vi "ReadAsyncErrorHandling.vi"(8 "ErrorIn":errorcluster, 11 "YActorIn":refnum<class "YActor.lvclass">) -> (0 "ErrorOut":errorcluster, 2 "AsyncErrorHandling":T1, 3 "YActorOut":refnum<class "YActor.lvclass">)   [LabVIEW 2021, in "YActor.lvclass"]
uses:
  YActor.lvclass
  AsyncErrorHandling.ctl
  YActor.lvclass/YActor.ctl
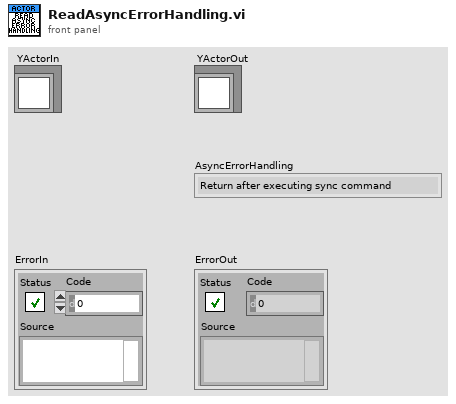
[diagram p1: front panel]
types:
  T1 = typedef "YActor.lvclass/AsyncErrorHandling.ctl" = enum16{"Return after executing sync command", "Return before executing sync command", "Don't return error"}
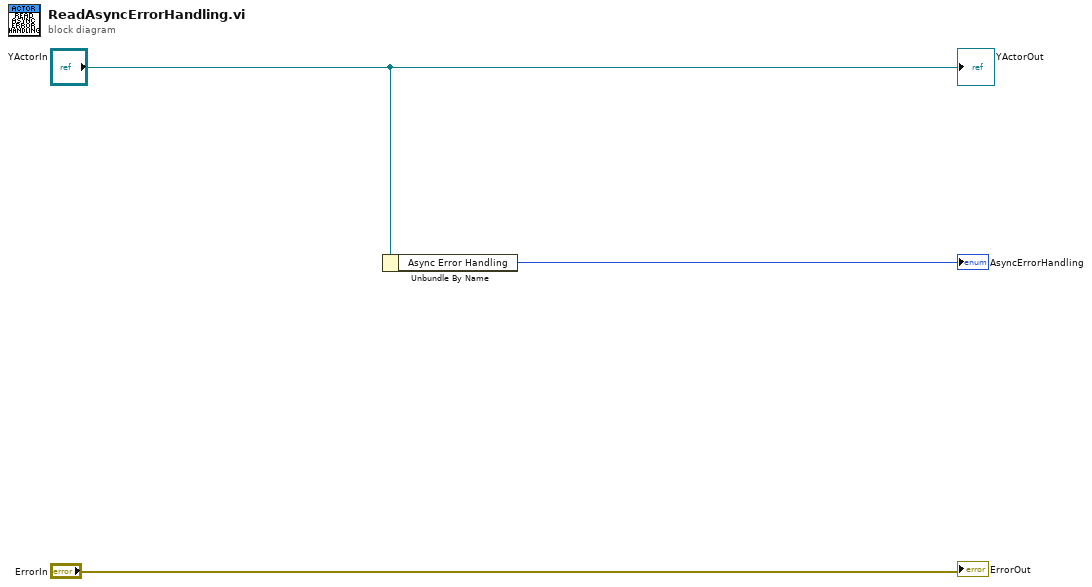
[diagram p0: block diagram]
diagram:
  n1 = Unbundle By Name("YActorIn") -> ("Async Error Handling"=→"AsyncErrorHandling":T1)
  "ErrorOut" <- "ErrorIn"
  "YActorOut" <- "YActorIn"
